vi "smart_gardner.vi"() -> ()   [LabVIEW 2022 SP3]
uses:
  <vilib>/Skyline/Tag/Shared/typedefs/DataType.ctl
  <vilib>/Skyline/Configuration/Configuration HTTP_class/Open Configuration API Key.vi
  <vilib>/Skyline/Tag/Wrapper/Wrapper_class/Write Tag (DBL).vi
  <vilib>/Skyline/Tag/Wrapper/Wrapper_class/Close Tag (Single).vi
  <vilib>/Skyline/Configuration/Configuration HTTP_class/NI Skyline Configuration HTTP.lvclass
  <vilib>/Skyline/Tag/Wrapper/Wrapper HTTP_class/NI Skyline Tag HTTP.lvclass
  <vilib>/Skyline/Tag/Wrapper/Wrapper_class/NI Skyline Tag.lvclass
  <vilib>/Skyline/Tag/Shared/NI Skyline Tag.lvlib
panel:
  out "Adjust Brightness":bool
  out "Adjust Temperature":bool
  out "Dispense Water":bool
  in  "Light":dbl
  in  "Temperature":dbl
  in  "Humidity":dbl
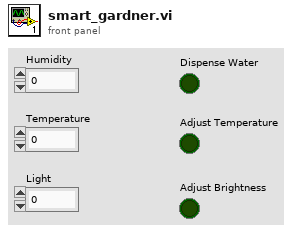
[diagram p1: front panel]
types:
  T1 = typedef "NI Skyline Tag.lvlib/DataType.ctl" = enum32{"Double", "I32", "String", "Boolean", "U64", "Timestamp"}
  T2 = enum16{"Start", "CheckHumidity", "CheckTemperature", "CheckLight", "AdjustHumidity", "AdjustTemperature", "AdjustLight", "Reset"}
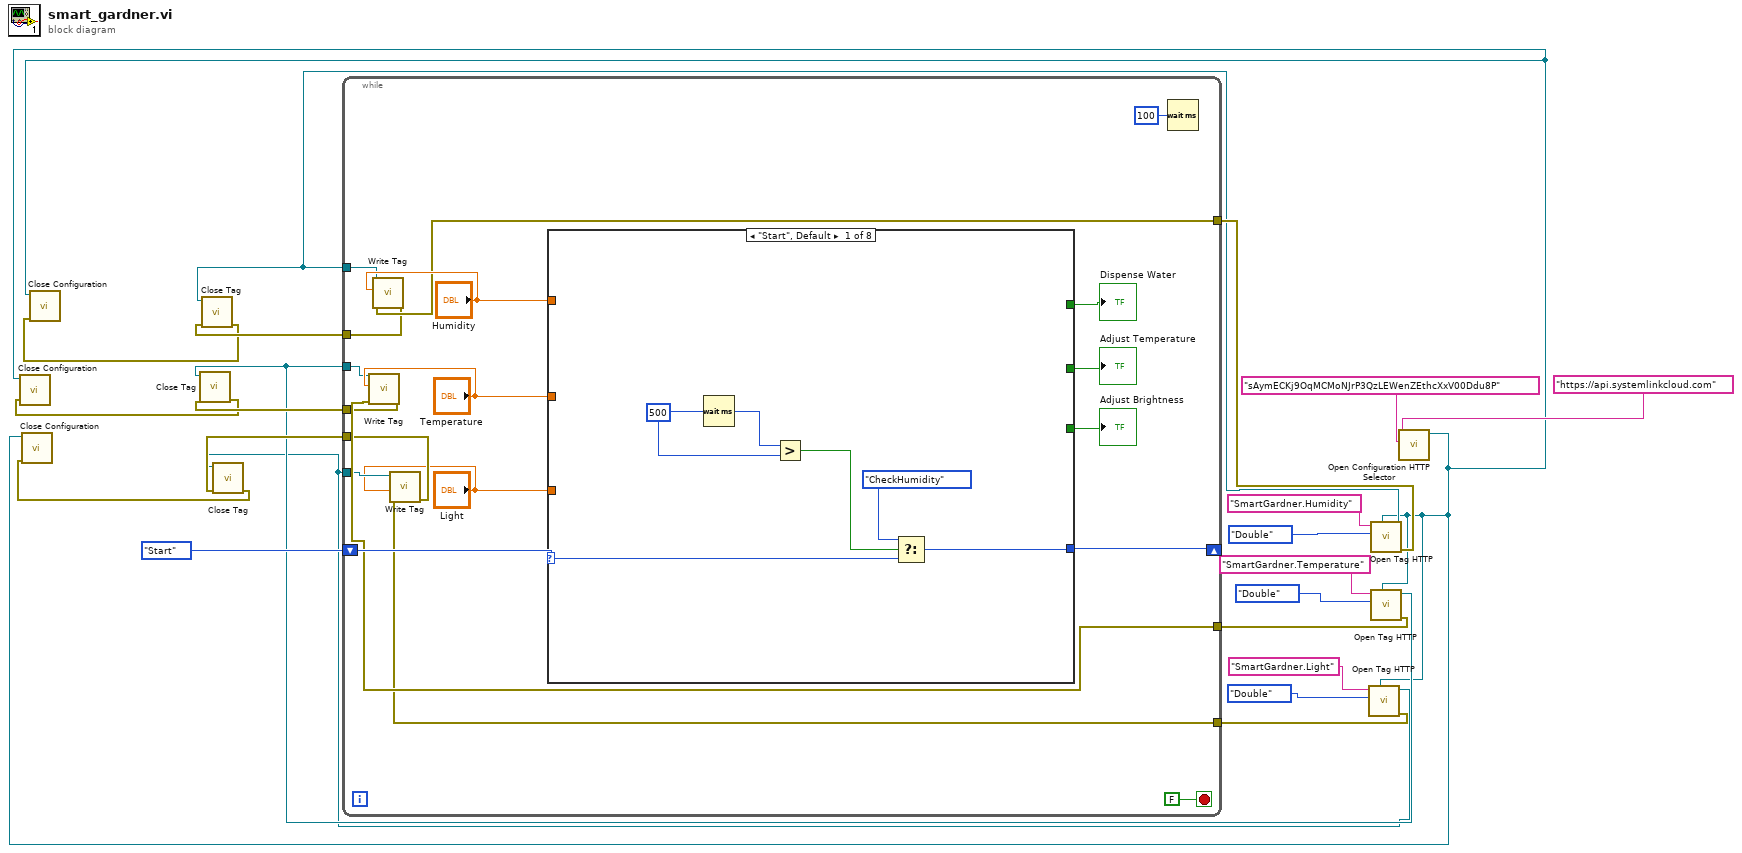
[diagram p0: block diagram]
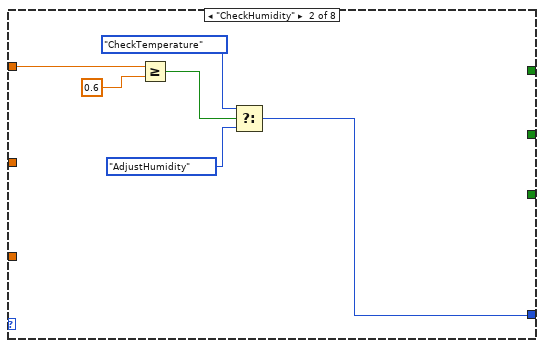
[diagram p2: hidden frame]
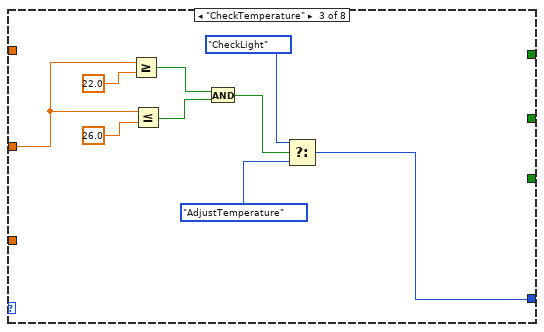
[diagram p3: hidden frame]
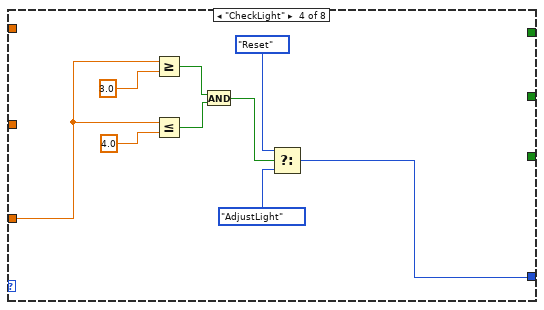
[diagram p4: hidden frame]
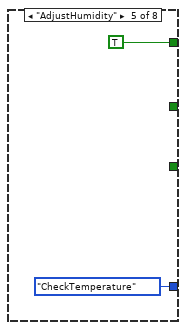
[diagram p5: hidden frame]
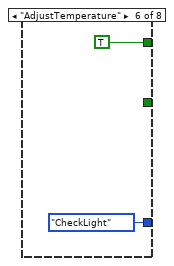
[diagram p6: hidden frame]
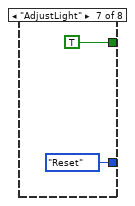
[diagram p7: hidden frame]
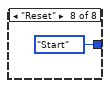
[diagram p8: hidden frame]
diagram:
  n1 = call-poly <vilib>:"Open Configuration HTTP Selector.vi"("api key"="sAymECKj9OqMCMoNJrP3QzLEWenZEthcXxV00Ddu8P", "server url"="https://api.systemlinkcloud.com") -> ("configuration"=w3:refnum<class "NI Skyline Configuration HTTP.lvclass">)  [unwired: 8 in, 1 out]
  n2 = call <vilib>:"Open Tag HTTP.vi"("configuration"=w3, "Data Type"=DataType."Double", "path"="SmartGardner.Light") -> ("error out"=w1:errorcluster, "tag"=w2:refnum<class "NI Skyline Tag.lvclass">)  [unwired: 7 in]
  n3 = call <vilib>:"Open Tag HTTP.vi"("configuration"=w3, "Data Type"=DataType."Double", "path"="SmartGardner.Humidity") -> ("error out"=w13:errorcluster, "tag"=w7:refnum<class "NI Skyline Tag.lvclass">)  [unwired: 7 in]
  n4 = call <vilib>:"Open Tag HTTP.vi"("configuration"=w3, "Data Type"=DataType."Double", "path"="SmartGardner.Temperature") -> ("error out"=w11:errorcluster, "tag"=w6:refnum<class "NI Skyline Tag.lvclass">)  [unwired: 7 in]
  n5 = while {
    shift-right: [w39] -> _
    shift-left: T2."Start" -> [w41]
    tunnel: w13 -> [w32]
    tunnel: [w31] -> w12
    tunnel: w11 -> [w30]
    tunnel: [w29] -> w10
    tunnel: [w28] -> w9
    tunnel: w7 -> [w27]
    tunnel: w6 -> [w26]
    tunnel: w2 -> [w25]
    tunnel: w1 -> [w24]
    stop <- FALSE stop-if-true
    n6 = call-poly <vilib>:"Write Tag.vi"("error in (no error)"=w30, "value"="Temperature", "tag in"=w26) -> ("error out"=w28:errorcluster)  [unwired: 7 in, 1 out]
    n7 = call-poly <vilib>:"Write Tag.vi"("error in (no error)"=w32, "value"="Humidity", "tag in"=w27) -> ("error out"=w31:errorcluster)  [unwired: 7 in, 1 out]
    n8 = call-poly <vilib>:"Write Tag.vi"("error in (no error)"=w24, "value"="Light", "tag in"=w25) -> ("error out"=w29:errorcluster)  [unwired: 7 in, 1 out]
    n9 = case shown="\"Start\", Default" w41 {
      selector: w41 -> [w43 _ _ _ _ _ _ _]
      tunnel: [w44 w48 w55 w63 T2."CheckTemperature" ("f") T2."CheckLight" ("f") T2."Reset" ("f") T2."Start" ("f")] -> w39
      tunnel: "Humidity" -> [_ w53 _ _ _ _ _ _]
      tunnel: "Temperature" -> [_ _ w54 _ _ _ _ _]
      tunnel: "Light" -> [_ _ _ w71 _ _ _ _]
      tunnel: [_ _ _ _ TRUE _ _ _] -> w38
      tunnel: [_ _ _ _ _ TRUE _ _] -> w37
      tunnel: [_ _ _ _ _ _ TRUE _] -> w36
      frame "Start", Default {
        w46 = u32 500 ("milliseconds to wait")
        n10 = Wait (ms)(milliseconds to wait=w46) -> (millisecond timer value=w47:u32)
        n11 = Greater?(x=w47, y=w46) -> (0:w45:bool)
        n12 = Select(t=T2."CheckHumidity", s=w45, f=w43) -> (s? t:f=w44:T2)
      }
      frame "CheckHumidity" {
        n13 = Greater Or Equal?(x=w53, y=0.6) -> (x >= y?=w51:bool)
        n14 = Select(t=T2."CheckTemperature", s=w51, f=T2."AdjustHumidity") -> (s? t:f=w48:T2)
      }
      frame "CheckTemperature" {
        n15 = Greater Or Equal?(x=w54, y=22.0) -> (x >= y?=w60:bool)
        n16 = Less Or Equal?(x=w54, y=26.0) -> (x <= y?=w59:bool)
        n17 = And(x=w60, y=w59) -> (x .and. y?=w58:bool)
        n18 = Select(t=T2."CheckLight", s=w58, f=T2."AdjustTemperature") -> (s? t:f=w55:T2)
      }
      frame "CheckLight" {
        n19 = Greater Or Equal?(x=w71, y=3.0) -> (x >= y?=w67:bool)
        n20 = Less Or Equal?(x=w71, y=4.0) -> (x <= y?=w68:bool)
        n21 = And(x=w67, y=w68) -> (x .and. y?=w66:bool)
        n22 = Select(t=T2."Reset", s=w66, f=T2."AdjustLight") -> (s? t:f=w63:T2)
      }
      frame "AdjustHumidity" {
      }
      frame "AdjustTemperature" {
      }
      frame "AdjustLight" {
      }
      frame "Reset" {
      }
    }
    "Dispense Water" <- w38
    "Adjust Temperature" <- w37
    "Adjust Brightness" <- w36
    n23 = Wait (ms)(milliseconds to wait=u32 100) -> ()  [unwired: 1 out]
  }
  n24 = call-poly <vilib>:"Close Tag.vi"("error in (no error)"=w9, "tag"=w6) -> ("error out"=w5:errorcluster)  [unwired: 9 in]
  n25 = call-dynamic "Close Configuration.vi"("error in (no error)"=w5, "configuration"=w3) -> ()  [unwired: 9 in, 1 out]
  n26 = call-poly <vilib>:"Close Tag.vi"("error in (no error)"=w12, "tag"=w7) -> ("error out"=w8:errorcluster)  [unwired: 9 in]
  n27 = call-dynamic "Close Configuration.vi"("error in (no error)"=w8, "configuration"=w3) -> ()  [unwired: 9 in, 1 out]
  n28 = call-poly <vilib>:"Close Tag.vi"("error in (no error)"=w10, "tag"=w2) -> ("error out"=w4:errorcluster)  [unwired: 9 in]
  n29 = call-dynamic "Close Configuration.vi"("error in (no error)"=w4, "configuration"=w3) -> ()  [unwired: 9 in, 1 out]
